vi "Punto_desplazado.vi"(10 "d":dbl, 11 "Zigma":dbl[](array[numeric])) -> (3 "Array out":dbl[](array[numeric]))   [LabVIEW 2011]
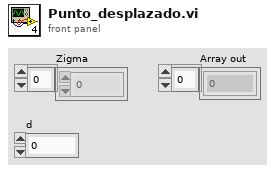
[diagram p1: front panel]
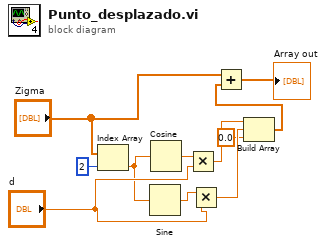
[diagram p0: block diagram]
diagram:
  n1 = Index Array(array="Zigma", index=2) -> (element=w7:dbl)
  n2 = Sine(x=w7) -> (sin(x)=w10:dbl)
  n3 = Cosine(x=w7) -> (cos(x)=w9:dbl)
  n4 = Multiply(x=w9, y="d") -> (x*y=w6:dbl)
  n5 = Multiply(x=w10, y="d") -> (x*y=w5:dbl)
  n6 = Build Array(w6, w5, 0.0 ("element")) -> (w3:dbl[])
  n7 = Add(x="Zigma", y=w3) -> (x+y=→"Array out":dbl[])
